vi "XLP80_EIP_ContUpdate.vi"(8 "err in":errorcluster) -> (0 "err out":errorcluster)   [LabVIEW 2021]
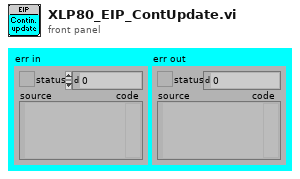
[diagram p1: front panel]
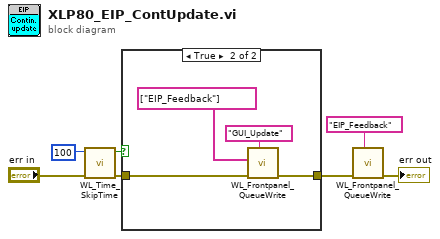
[diagram p0: block diagram]
diagram:
  n1 = call "WL_Time_SkipTime.vi"("err in"="err in", "SkipTime[ms]"=u32 100) -> ("err out"=w5:errorcluster, "Run"=w4:bool)  [unwired: 8 in]
  n2 = case shown="True" w4 {
    tunnel: [w8 w9] -> w2
    tunnel: w5 -> [w8 w10]
    frame False {
    }
    frame True {
      n3 = call "WL_Frontpanel_QueueWrite.vi"("Command (error only)"="GUI_Update", "err in"=w10, "Parameters"=string[] ["EIP_Feedback"]) -> ("err out"=w9:errorcluster)  [unwired: 8 in]
    }
  }
  n4 = call "WL_Frontpanel_QueueWrite.vi"("Command (error only)"="EIP_Feedback", "err in"=w2) -> ("err out"=→"err out":errorcluster)  [unwired: 9 in]
